vi "Get ECAT IOVar VS refs.vi"(8 "Fehler (Eingang, kein Fehler)":errorcluster, 9 "Section Name":string, 10 "Item Ref":T1 format="%.0x", 11 "I/O Variable Data in":T2[](array[typedef]) {"VS ref" format="%.0x"}) -> (0 "Fehler (Ausgang)":errorcluster, 2 "Channel Refs":T1[](array[typedef]) format="%.0x", 3 "I/O Variable Data out":T2[](array[typedef]) {"VS ref" format="%.0x"})   [LabVIEW 2016, in "Scan Engine Custom Device.lvlib"]
uses:
  Scan Engine Custom Device.lvlib
  <vilib>/NI Veristand/Custom Device API/Custom Device Item Ref.ctl
  Type Defs/Generic ECAT Slave IOV Cluster.ctl
  Type Defs/UDV Data Type.ctl
  <vilib>/NI Veristand/Custom Device API/Custom Device API.lvlib
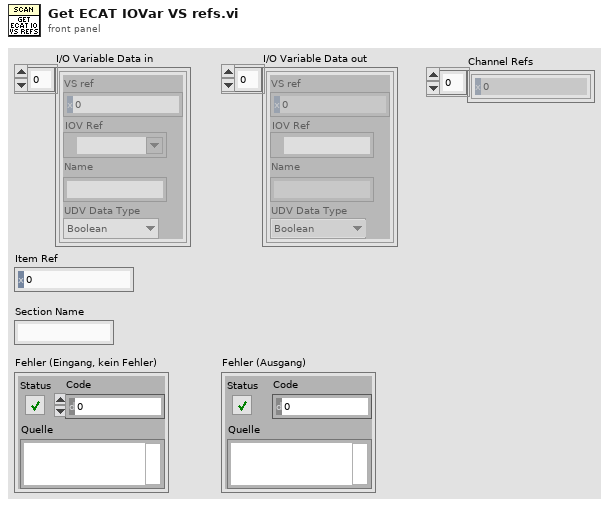
[diagram p1: front panel]
types:
  T1 = typedef "Custom Device API.lvlib/Custom Device Item Ref.ctl" = u64
  T2 = typedef "Scan Engine Custom Device.lvlib/Generic ECAT Slave IOV Cluster.ctl" = cluster{"VS ref":T1, "IOV Ref":refnum<k21>, "Name":string, "UDV Data Type":T3}
  T3 = typedef "Scan Engine Custom Device.lvlib/UDV Data Type.ctl" = enum16{"Boolean", "Fixed Point", "Int8", "Int16", "Int32", "Int64", "U32 Bit Field", "UInt8", "UInt16", "UInt32", "UInt64", "Other"}
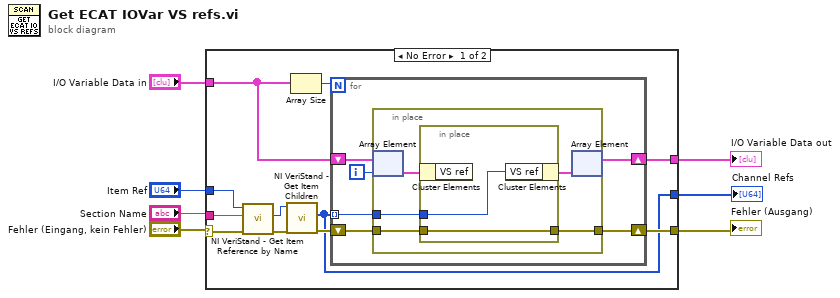
[diagram p0: block diagram]
diagram:
  n1 = case shown="No Error" "Fehler (Eingang, kein Fehler)" {
    selector: "Fehler (Eingang, kein Fehler)" -> [w12 w33]
    tunnel: "Item Ref" -> [w18 _]
    tunnel: [w9 w32] -> w6
    tunnel: [w17 w33] -> w5
    tunnel: "I/O Variable Data in" -> [w10 w32]
    tunnel: "Section Name" -> [w11 _]
    tunnel: [w8 _] -> w1
    frame No Error {
      n2 = call <vilib>:"NI VeriStand - Get Item Reference by Name.vi"("error in (no error)"=w12, "Item Name"=w11, "Parent Ref in"=w18) -> ("error out"=w14:errorcluster, "Item Ref"=w13:T1)  [unwired: 5 in, 2 out]
      n3 = call <vilib>:"NI VeriStand - Get Item Children.vi"("error in (no error)"=w14, "Item Ref in"=w13) -> ("error out"=w15:errorcluster, "Child Refs"=w8:T1[])  [unwired: 6 in, 2 out]
      n4 = Array Size(array=w10) -> (size(s)=w16:i32)
      n5 = for {
        N: w16 -> [_]
        tunnel: w8 -> [w22] mode=indexing
        shift-right: [w21] -> w9
        shift-left: w10 -> [w24]
        shift-right: [w19] -> w17
        shift-left: w15 -> [w23]
        i -> [w20]
        n6 = in-place {
          in-place-border: w23 -> [w26]
          in-place-border: w22 -> [w28]
          in-place-border: [w25] -> w19
          n7 = in-place-array #1(w24, w20) -> (w29:T2)
          n8 = in-place {
            in-place-border: w28 -> [w30]
            in-place-border: [w31] -> w25
            in-place-border: w26 -> [w31]
            n9 = in-place-cluster #2(w29) -> ()  [unwired: 1 out]
            n10 = in-place-cluster #2("VS ref"=w30) -> (w27:T2)
          }
          n11 = in-place-array #1(w27) -> (w21:T2[])  [unwired: 1 out]
        }
      }
    }
    frame Error {
    }
  }
  "I/O Variable Data out" <- w6
  "Fehler (Ausgang)" <- w5
  "Channel Refs" <- w1
